vi "Available Workers.vi"(7 "Refresh? (F)":bool) -> (2 "Workers Map":map{string, T1}(c390), 3 "Names":string[](array[string]))   [LabVIEW 2022 SP3, in "FlexBlocks Support.lvlib"]
uses:
  FlexBlocks Support.lvlib
  Worker Info.ctl
  <vilib>/picture/picture.llb/imagedata.ctl
  Worker Variant.ctl
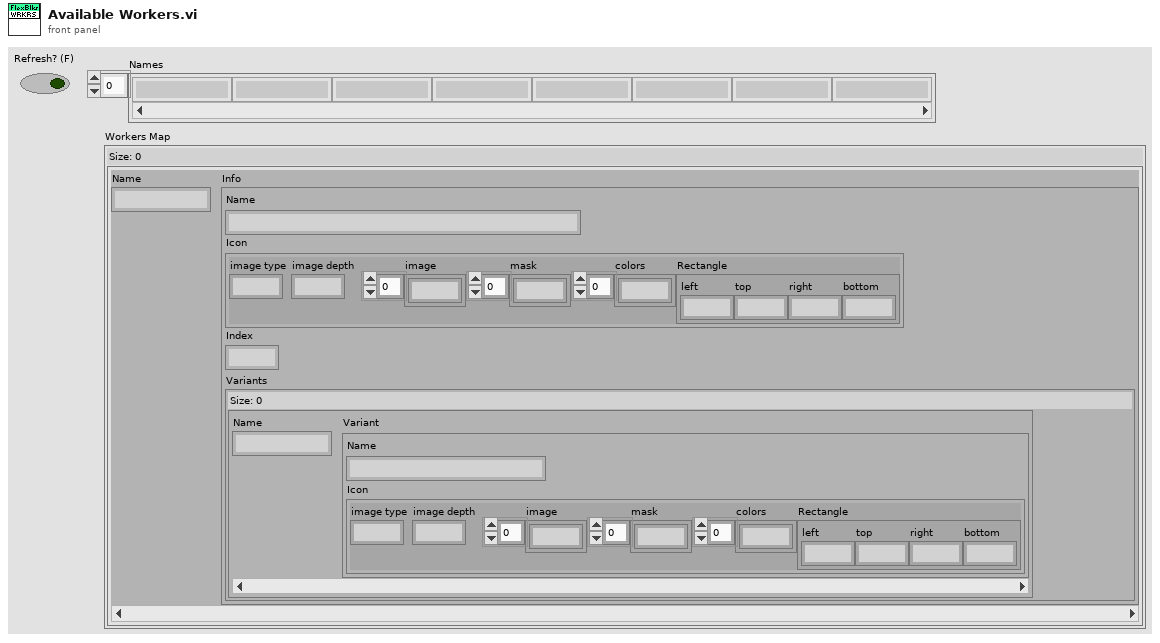
[diagram p1: front panel]
types:
  T1 = typedef "FlexBlocks Support.lvlib/Worker Info.ctl" = cluster{"Name":string, "Icon":T2, "Index":i32, "Variants":map{string, T3}}
  T2 = typedef "imagedata.ctl" = cluster{"image type":i32, "image depth":i32, "image":u8[], "mask":u8[], "colors":u32[], "Rectangle":cluster{"left":i16, "top":i16, "right":i16, "bottom":i16}}
  T3 = typedef "FlexBlocks Support.lvlib/Worker Variant.ctl" = cluster{"Name":string, "Icon":T2}
  T4 = typedef "FlexBlocks Support.lvlib/Paths.ctl" = cluster{"FlexBlocks":path, "Workers Root":path, "Specialized Editors":path, "Worker Template":path, "SM Template":path, "Read Control Value Vim":path, "Write Indicator Value Vim":path}
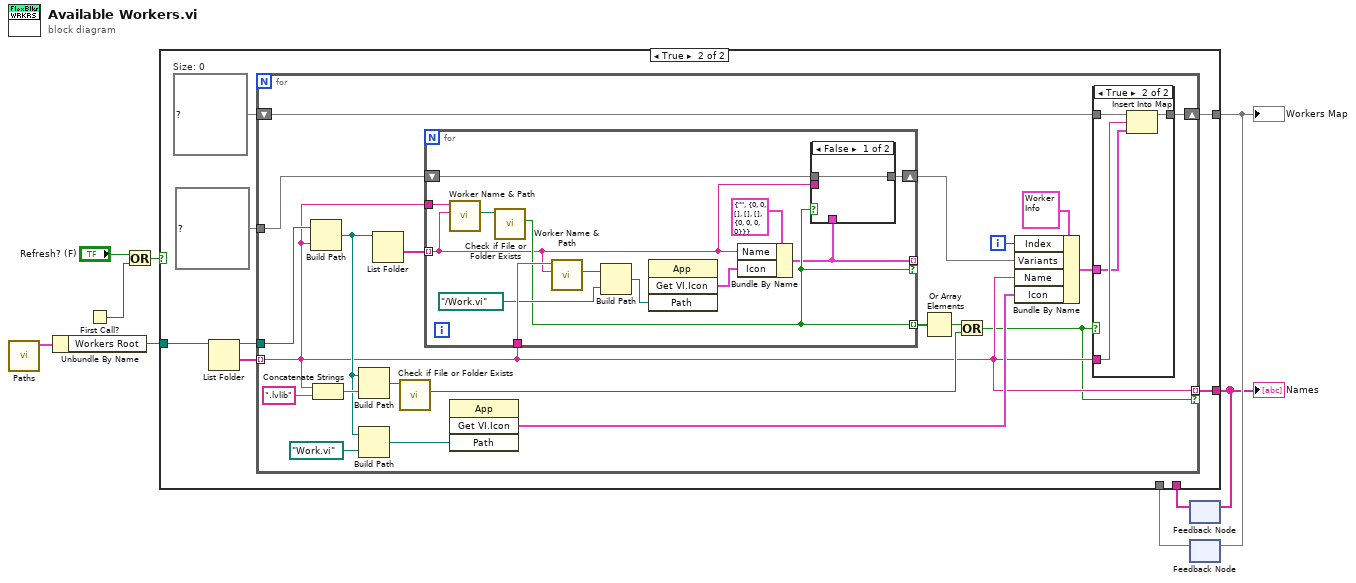
[diagram p0: block diagram]
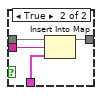
[diagram p3: hidden frame]
diagram:
  n1 = call "Paths.vi"() -> ("Paths"=w5:T4)  [unwired: 11 in]
  n2 = Unbundle By Name(w5) -> ("Workers Root"=w4:path)
  n3 = First Call?() -> (First Call?: T/F=w8:bool)
  n4 = Or(x="Refresh? (F)", y=w8) -> (x .or. y?=w7:bool)
  n5 = feedback #1() -> (w1:string[])  [unwired: 1 in]
  n6 = feedback #2() -> (w6:map{string, T1})  [unwired: 1 in]
  n7 = case shown="True" w7 {
    tunnel: w4 -> [_ w18]
    tunnel: w6 -> [w11 _]
    tunnel: [w11 w14] -> w3
    tunnel: [w10 w13] -> w2
    tunnel: w1 -> [w10 _]
    frame False {
    }
    frame True {
      w15 = map{string, T1} {}  # Size: 0
      n8 = List Folder(path=w18) -> (path out=w16:path, folder names=w17:string[])  [unwired: 3 in, 2 out]
      n9 = for {
        tunnel: w17 -> [w22] mode=indexing
        tunnel: w16 -> [w39]
        shift-right: [w29] -> w14
        shift-left: w15 -> [w31]
        tunnel: [w22] -> w13 mode=indexing if=w21
        tunnel: map{string, T3} {} ("Variants") -> [w20]
        i -> [w23]
        n10 = Build Path(base path=w39, name or relative path=w22) -> (appended path=w27:path)
        n11 = Concatenate Strings(w22, ".lvlib" ("string")) -> (w37:string)
        n12 = Build Path(base path=w27, name or relative path=w37) -> (appended path=w36:path)
        n13 = Build Path(base path=w27, name or relative path=path "Work.vi") -> (appended path=w25:path)
        n14 = List Folder(path=w27) -> (folder names=w34:string[])  [unwired: 3 in, 3 out]
        n15 = call <vilib>:"Check if File or Folder Exists.vi"("path"=w36) -> ("file or folder exists?"=w35:bool)  [unwired: 8 in, 2 out]
        n16 = for {
          tunnel: w34 -> [w40] mode=indexing
          tunnel: w22 -> [w52]
          tunnel: [w41] -> _ mode=indexing if=w42
          tunnel: [w42] -> w33 mode=indexing
          tunnel: w22 -> [w49]
          shift-right: [w44] -> w19
          shift-left: w20 -> [w43]
          n17 = call "Worker Name & Path.vi"("Variant"=w40, "Worker"=w52) -> ("lvlib Path"=w51:path)  [unwired: 5 in, 4 out]
          n18 = call <vilib>:"Check if File or Folder Exists.vi"("path"=w51) -> ("file or folder exists?"=w42:bool)  [unwired: 8 in, 2 out]
          n19 = call "Worker Name & Path.vi"("Variant"=w40, "Worker"=w49) -> ("lvlib Path"=w48:path)  [unwired: 5 in, 4 out]
          n20 = Build Path(base path=w48, name or relative path=path "../Work.vi") -> (appended path=w46:path)
          n21 = invoke class="App" method="Get VI.Icon"("Path"=w46) -> ("Get VI.Icon"=w45:T2)  [unwired: 3 in, 3 out]
          n22 = Bundle By Name(cluster=T3 {"Name"="", "Icon"={"image type"=0, "image depth"=0, "image"=[], "mask"=[], "colors"=[], "Rectangle"={"left"=0, "top"=0, "right"=0, "bottom"=0}}} ("Worker Variant"), "Name"=w40, "Icon"=w45) -> (w41:T3)
          n23 = case shown="False" w42 {
            tunnel: [w53 w57] -> w44
            tunnel: w43 -> [w53 w56]
            tunnel: w41 -> [_ w55]
            tunnel: w40 -> [_ w54]
            frame False {
            }
            frame True {
              n24 = Insert Into Map(map in=w56, key=w54, value=w55) -> (map out=w57:map{string, T3})  [unwired: 2 out]
            }
          }
        }
        n25 = invoke class="App" method="Get VI.Icon"("Path"=w25) -> ("Get VI.Icon"=w24:T2)  [unwired: 3 in, 3 out]
        n26 = Or Array Elements(Boolean array=w33) -> (logical OR=w32:bool)
        n27 = Or(x=w32, y=w35) -> (x .or. y?=w21:bool)
        n28 = Bundle By Name(cluster=T1 {"Name"="", "Icon"={"image type"=0, "image depth"=0, "image"=[], "mask"=[], "colors"=[], "Rectangle"={"left"=0, "top"=0, "right"=0, "bottom"=0}}, "Index"=0, "Variants"={}} ("Worker Info"), "Index"=w23, "Variants"=w19, "Name"=w22, "Icon"=w24) -> (w28:T1)
        n29 = case shown="True" w21 {
          tunnel: w31 -> [w58 w62]
          tunnel: [w58 w59] -> w29
          tunnel: w28 -> [_ w60]
          tunnel: w22 -> [_ w61]
          frame False {
          }
          frame True {
            n30 = Insert Into Map(map in=w62, key=w61, value=w60) -> (map out=w59:map{string, T1})  [unwired: 2 out]
          }
        }
      }
    }
  }
  "Workers Map" <- w3
  "Names" <- w2
  n31 = feedback-in #1(w2) -> ()
  n32 = feedback-in #2(w3) -> ()
